vi "Position Single Button OK Button.vi"(8 "error in (no error)":errorcluster, 10 "Message":refnum<vi>, 11 "Button Ref":refnum<vi>) -> (0 "error out":errorcluster)   [LabVIEW 2014]
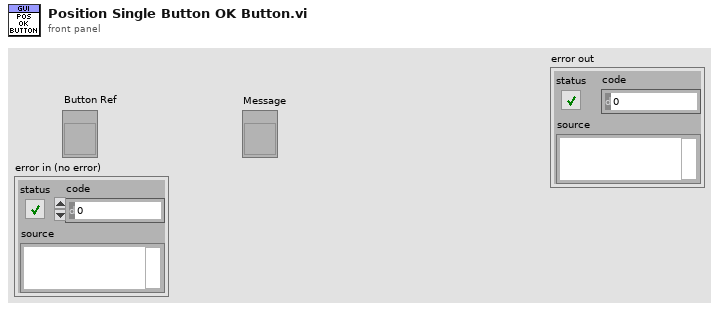
[diagram p1: front panel]
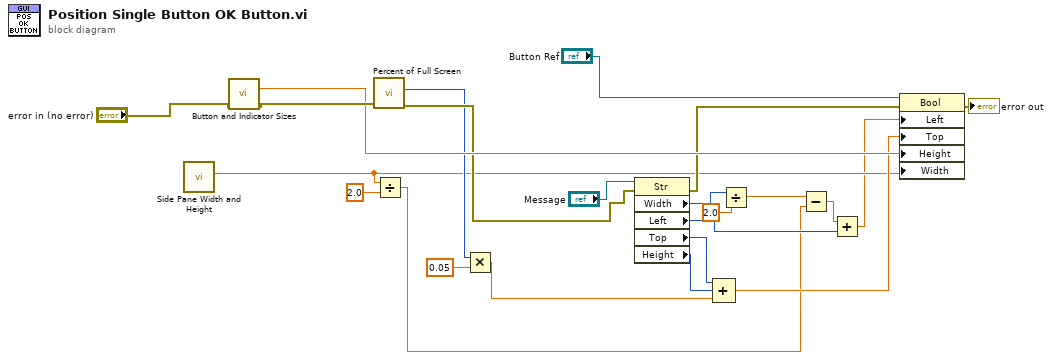
[diagram p0: block diagram]
diagram:
  n1 = call "Side Pane Width and Height.vi"() -> ("Width"=w9:dbl)  [unwired: 9 in, 2 out]
  n2 = call "Button and Indicator Sizes.vi"("error in (no error)"="error in (no error)") -> ("Button Height"=w19:dbl, "error out"=w21:errorcluster)  [unwired: 10 in, 3 out]
  n3 = call "Percent of Full Screen.vi"("error in (no error)"=w21) -> ("error out"=w17:errorcluster, "Bottom"=w12:i16)  [unwired: 8 in, 1 out]
  n4 = Divide(x=w9, y=2.0) -> (x/y=w3:dbl)
  n5 = Multiply(x=w12, y=0.05) -> (x*y=w10:dbl)
  n6 = property class="Str"(reference="Message", error in=w17) -> (error out=w16:errorcluster, "Width"=w6:u32, "Left"=w7:i32, "Top"=w15:i32, "Height"=w14:u32)  [unwired: 1 out]
  n7 = Compound Arithmetic op=ADD(w15, w14, w10) -> (w13:dbl)
  n8 = Divide(x=w6, y=2.0) -> (x/y=w4:dbl)
  n9 = Subtract(x=w4, y=w3) -> (x-y=w2:dbl)
  n10 = Add(x=w2, y=w7) -> (x+y=w1:dbl)
  n11 = property class="Bool"(reference="Button Ref", error in=w16, "Left"=w1, "Top"=w13, "Height"=w19, "Width"=w9) -> (error out=→"error out":errorcluster)  [unwired: 1 out]
